vi "AlGaInPAs_prep_run_disc_v04.vi"(2 "Debug Mode":bool, 3 "Elapsed Time(s)":dbl, 4 "State":enum16{"Edit", "Start", "Run", "End", "Idle"}(ring), 5 "Argument List In":string[](array[string])) -> (0 "Status Out":string, 1 "Argument List Out":string[](array[string]))   [LabVIEW 2011]
panel:
  out "total time":dbl
  out "is OK?":bool
  out "Run started?":bool
  out "AsH3?":bool
  out "PH3?":bool
  out "In?":bool
  out "Ga?":bool
  out "Al?":bool
  in  "Prep As":bool caption="Pre-run"
  in  "Prep P":bool caption="Pre-run"
  in  "Prep In":bool caption="Pre-run"
  in  "Prep Ga":bool caption="Pre-run"
  in  "run_time":dbl caption="run time (s)"
  in  "prep_time":dbl caption="pre-run time (s)"
  in  "Prep Al":bool caption="Pre-run"
  in  "Run As":bool caption="Run"
  in  "AsH3 Flow":dbl caption="AsH3 Flow (0-10 sccm)" format="%.2f"
  in  "P Flow":dbl caption="P Flow (0-100 sccm)" format="%.2f"
  in  "Run P":bool caption="Run"
  in  "In Flow":dbl caption="In Flow (0-100 sscm)" format="%.2f"
  in  "Run In":bool caption="Run"
  in  "Run Ga":bool caption="Run"
  in  "Ga Flow":dbl caption="Ga Flow (0-10 sscm)" format="%.2f"
  in  "Run Al":bool caption="Run"
  in  "Al Flow":dbl caption="Al Flow (0-100 sscm)" format="%.2f"
  in  "Cancel":bool
  in  "OK":bool
  out "tTotal(s) 2":dbl
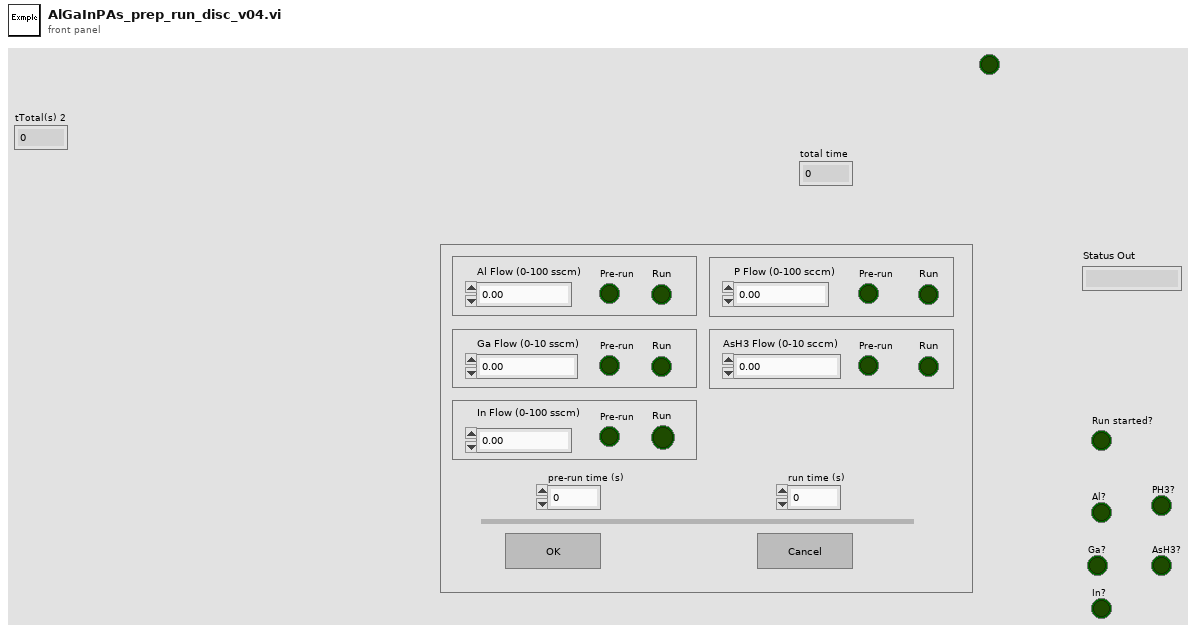
[diagram p1: front panel]
types:
  T1 = enum16{"Discrete", "Continuous", "Instantaneous"}
  T2 = enum32{"Invalid", "Default", "Floating", "Floating/Auto-Hide", "Modal"}
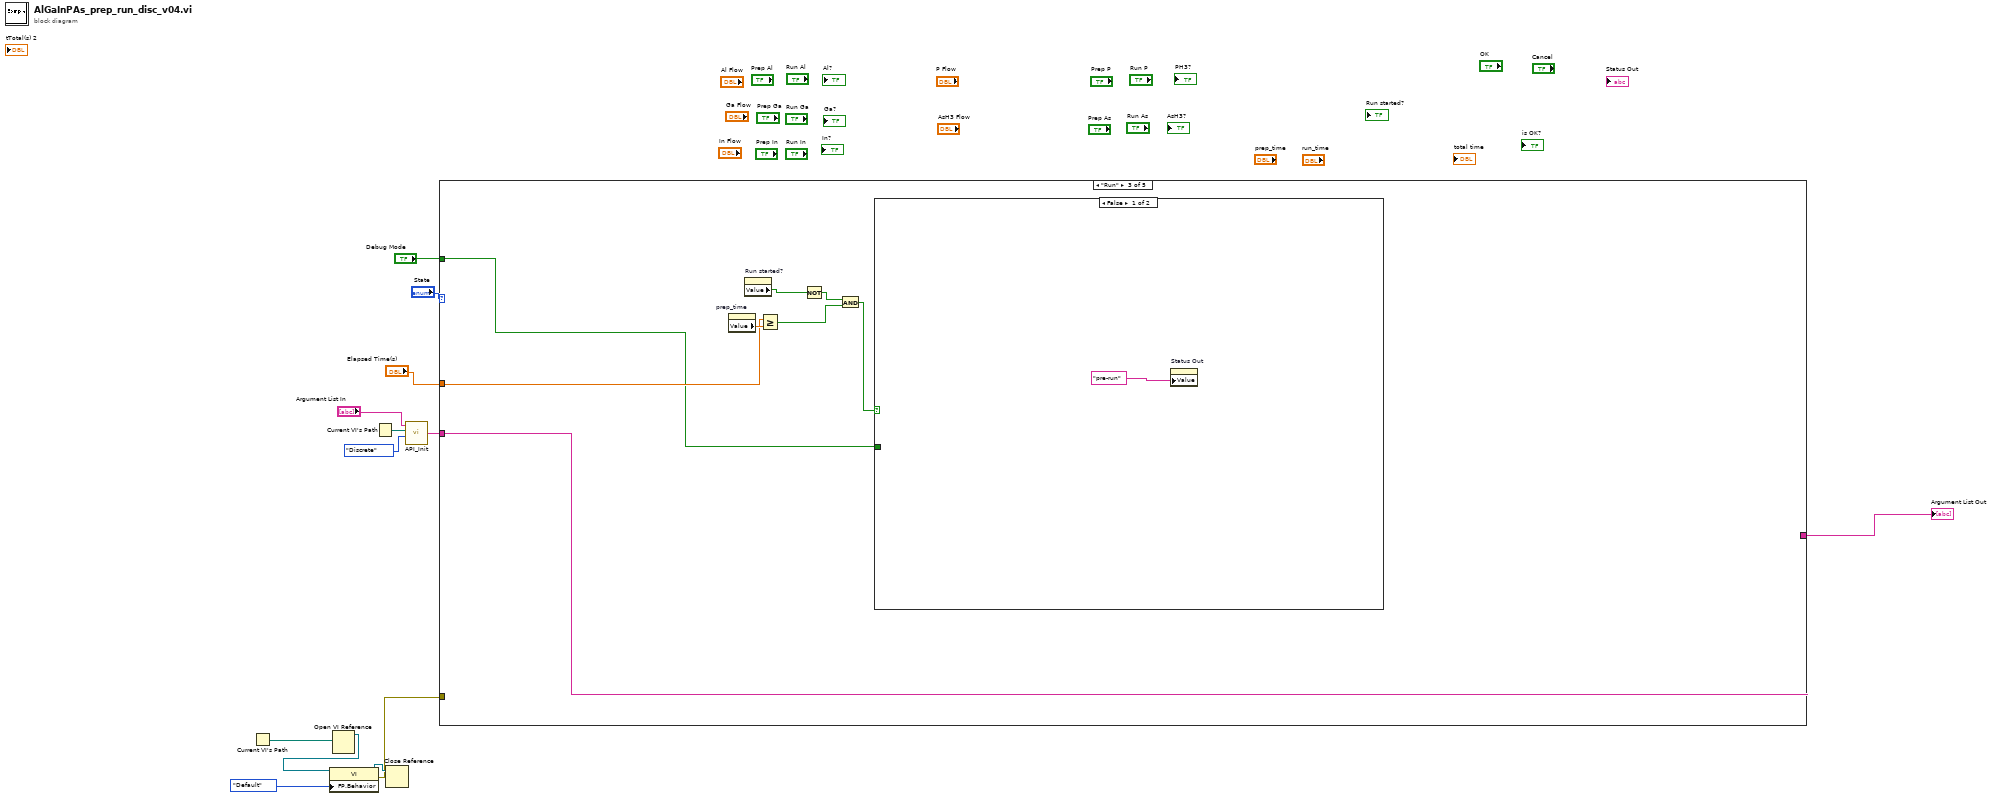
[diagram p0: block diagram]
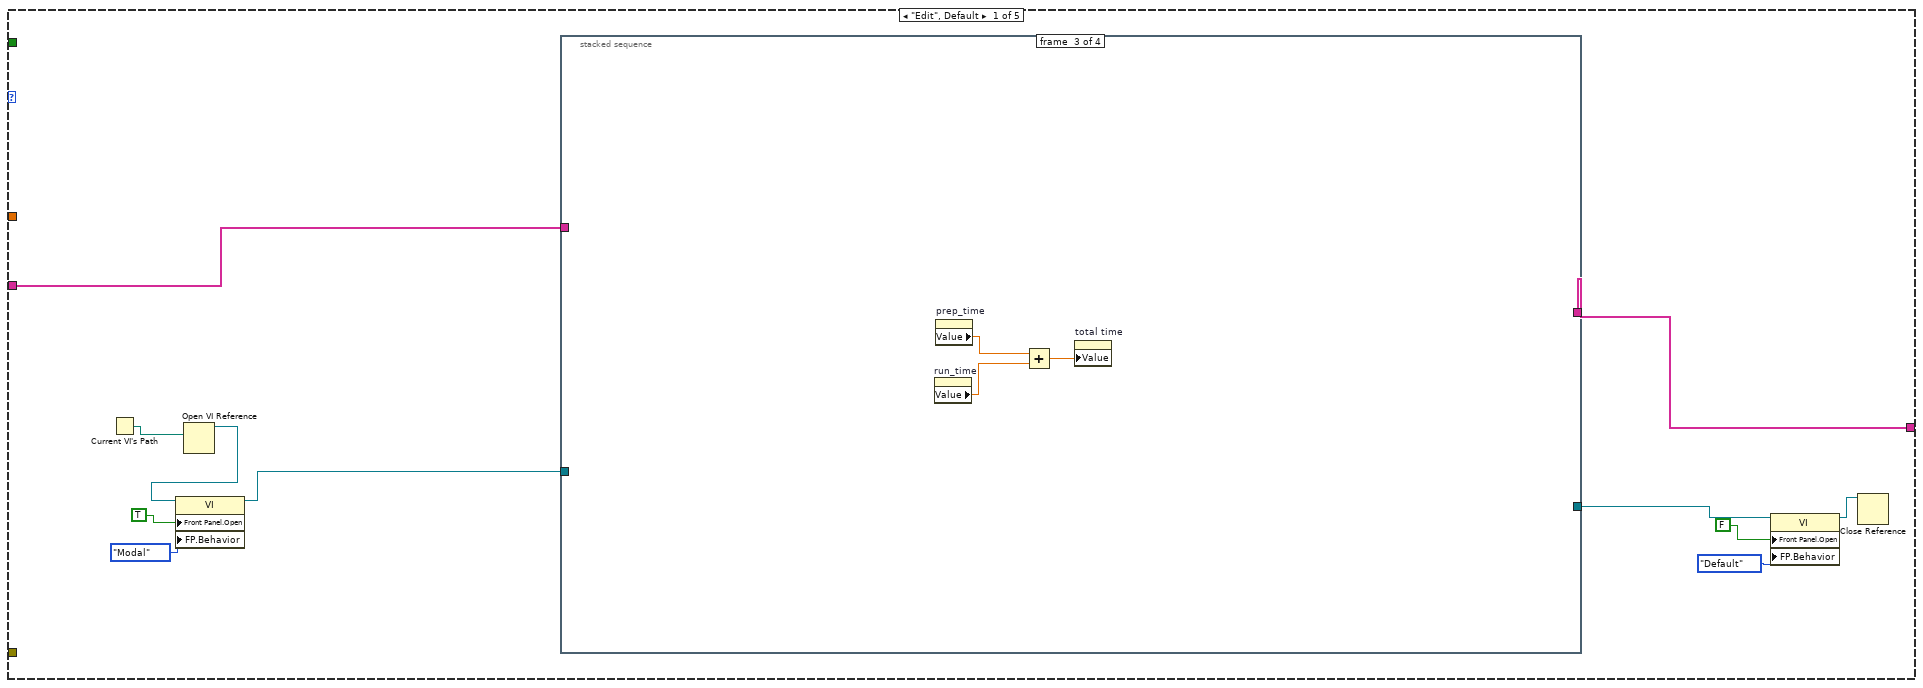
[diagram p2: hidden frame]
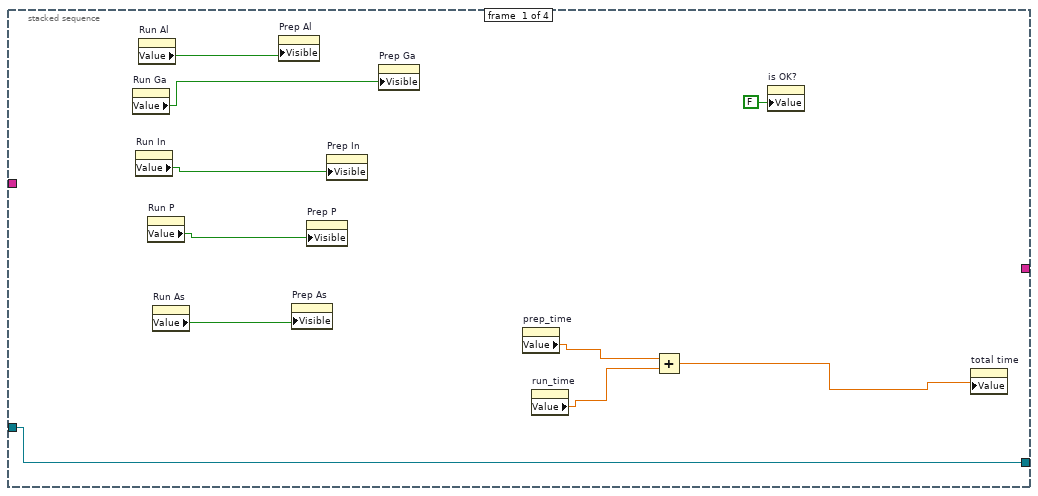
[diagram p3: hidden frame]
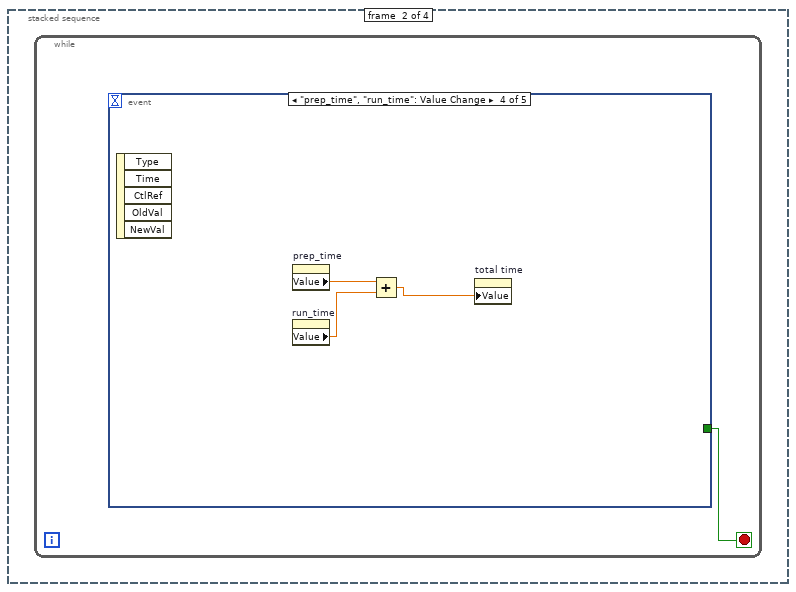
[diagram p4: hidden frame]
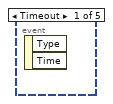
[diagram p5: hidden frame]
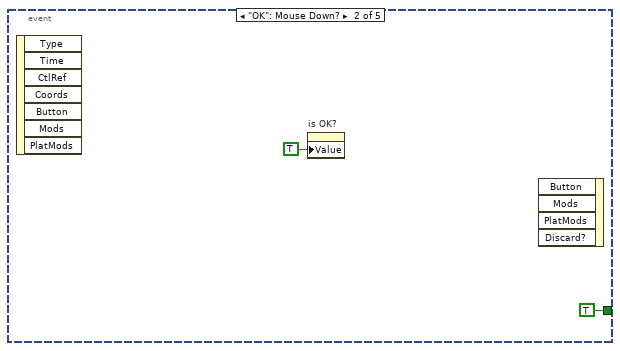
[diagram p6: hidden frame]
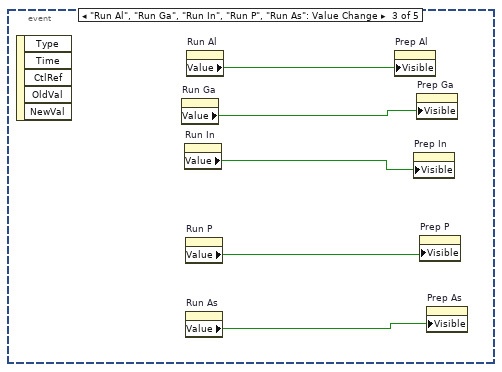
[diagram p7: hidden frame]
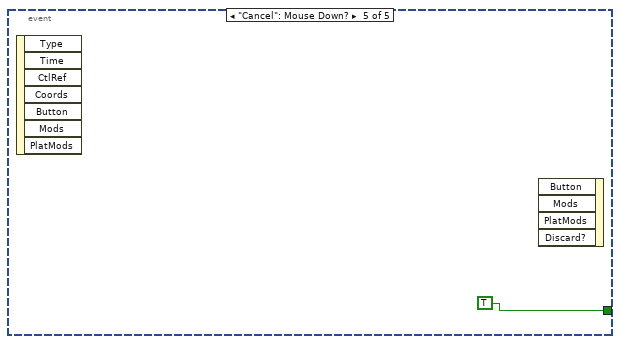
[diagram p8: hidden frame]
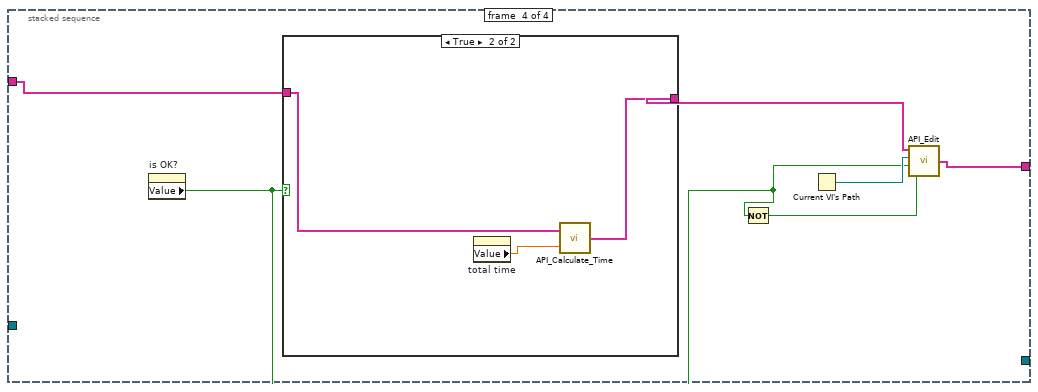
[diagram p9: hidden frame]
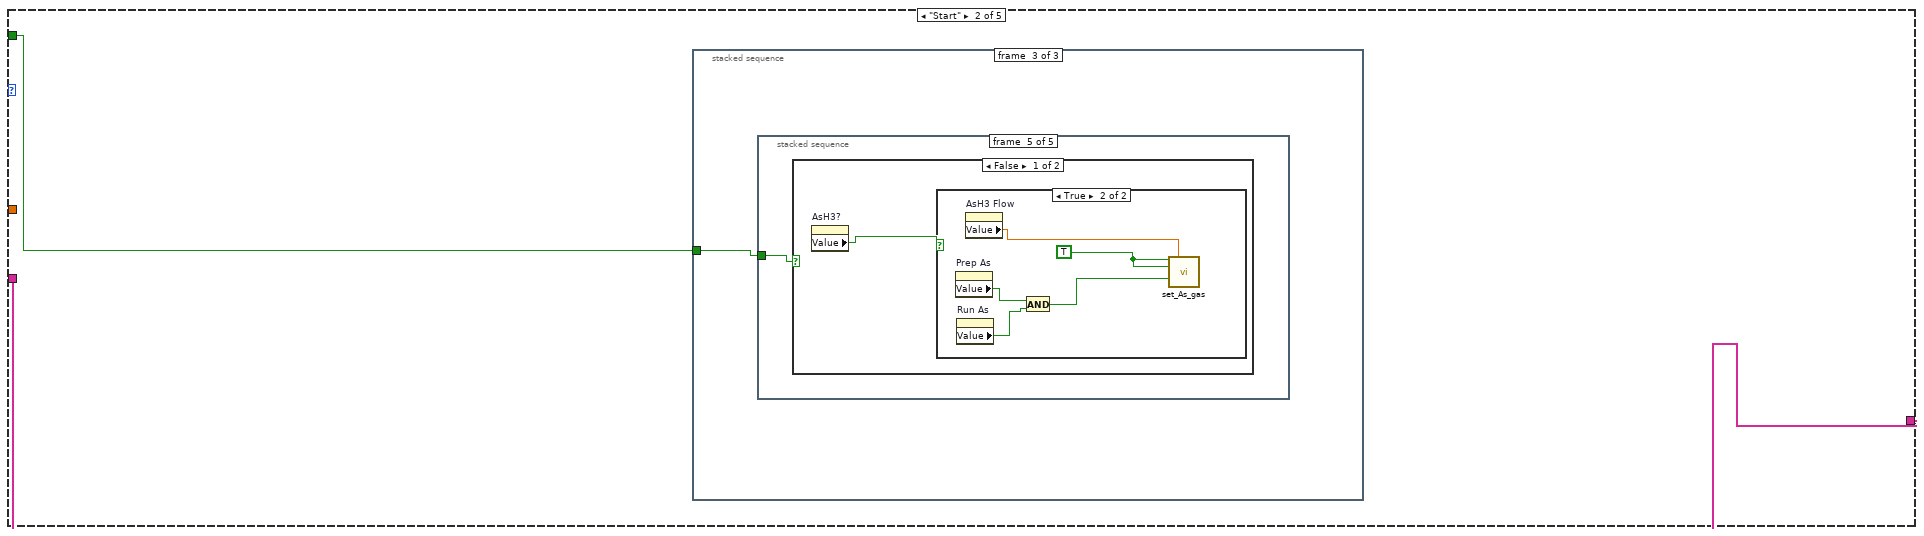
[diagram p11: hidden frame]
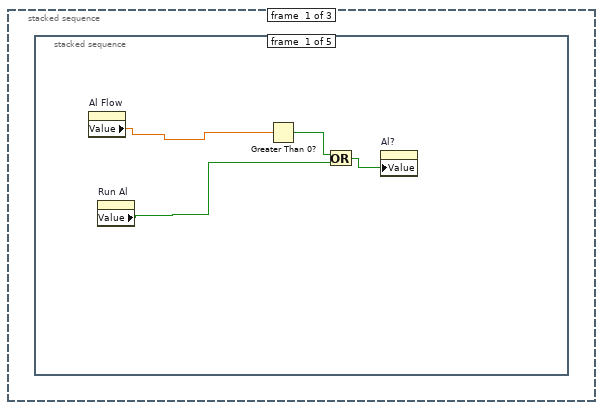
[diagram p12: hidden frame]
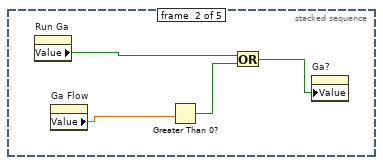
[diagram p13: hidden frame]
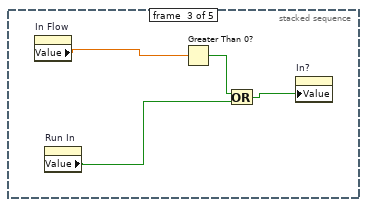
[diagram p14: hidden frame]
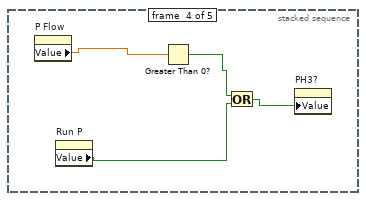
[diagram p15: hidden frame]
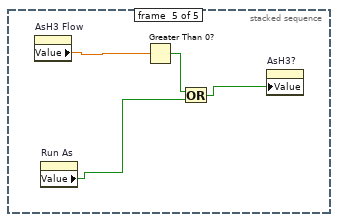
[diagram p16: hidden frame]
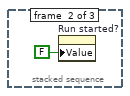
[diagram p17: hidden frame]
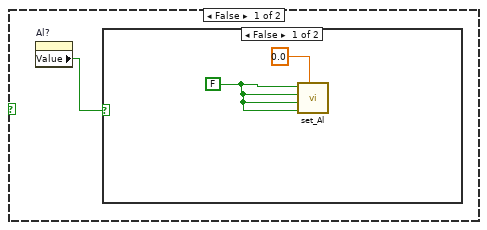
[diagram p19: hidden frame]
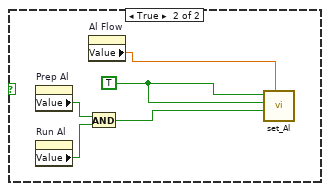
[diagram p20: hidden frame]
diagram:
  n1 = Current VI's Path() -> (path=w9:path)
  n2 = Open VI Reference(vi path=w9) -> (vi reference=w8:refnum<vi>)  [unwired: 1 in, 5 out]
  n3 = property class="VI"(reference=w8, "FP.Behavior"=T2."Default" ("Front Panel Window:Behavior")) -> (reference out=w6:refnum<vi>, error out=w5:errorcluster)  [unwired: 1 in]
  n4 = Current VI's Path() -> (path=w4:path)
  n5 = Close Reference(reference=w6) -> ()  [unwired: 1 in, 1 out]
  n6 = call "API_Init.vi"("API Mode"=T1."Discrete", "VI Path"=w4, "Argument List In"="Argument List In") -> ("Argument List Out"=w1:string[])  [unwired: 1 in]
  n7 = case shown="\"Run\"" "State" {
    tunnel: "Debug Mode" -> [_ w60 w134 _ _]
    tunnel: "Elapsed Time(s)" -> [_ _ w135 _ _]
    tunnel: w1 -> [w15 w61 w137 w179 w180]
    tunnel: [w14 w61 w137 w179 w180] -> w10
    tunnel: w5 -> [_ _ _ _ _]
    frame "Edit", Default {
      n8 = Current VI's Path() -> (path=w20:path)
      n9 = Open VI Reference(vi path=w20) -> (vi reference=w19:refnum<vi>)  [unwired: 1 in, 5 out]
      n10 = property class="VI"(reference=w19, "Front Panel.Open"=TRUE ("Front Panel Window:Open"), "FP.Behavior"=T2."Modal" ("Front Panel Window:Behavior")) -> (reference out=w18:refnum<vi>)  [unwired: 1 in, 1 out]
      n11 = stacked-sequence {
        tunnel: w15 -> [_ _ _ w53]
        tunnel: w18 -> [w32 _ _ _]
        tunnel: [w32 _ _ _] -> w22
        tunnel: [_ _ _ w51] -> w14
        frame #0 {
          n12 = property on="Run Ga" class="Bool (strict)"() -> ("Value"=w28:bool)  [unwired: 2 in, 2 out]
          n13 = property on="Run In" class="Bool (strict)"() -> ("Value"=w27:bool)  [unwired: 2 in, 2 out]
          n14 = property on="Run Al" class="Bool (strict)"() -> ("Value"=w29:bool)  [unwired: 2 in, 2 out]
          n15 = property on="Run P" class="Bool (strict)"() -> ("Value"=w26:bool)  [unwired: 2 in, 2 out]
          n16 = property on="Run As" class="Bool (strict)"() -> ("Value"=w25:bool)  [unwired: 2 in, 2 out]
          n17 = property on="Prep Al" class="Bool (strict)"("Visible"=w29) -> ()  [unwired: 2 in, 2 out]
          n18 = property on="Prep As" class="Bool (strict)"("Visible"=w25) -> ()  [unwired: 2 in, 2 out]
          n19 = property on="Prep P" class="Bool (strict)"("Visible"=w26) -> ()  [unwired: 2 in, 2 out]
          n20 = property on="Prep In" class="Bool (strict)"("Visible"=w27) -> ()  [unwired: 2 in, 2 out]
          n21 = property on="Prep Ga" class="Bool (strict)"("Visible"=w28) -> ()  [unwired: 2 in, 2 out]
          n22 = property on="prep_time" class="DigNum (strict)"() -> ("Value"=w34:dbl)  [unwired: 2 in, 2 out]
          n23 = property on="run_time" class="DigNum (strict)"() -> ("Value"=w33:dbl)  [unwired: 2 in, 2 out]
          n24 = Add(x=w34, y=w33) -> (x+y=w30:dbl)
          n25 = property on="is OK?" class="Bool (strict)"("Value"=FALSE ("is OK?")) -> ()  [unwired: 2 in, 2 out]
          n26 = property on="total time" class="DigNum (strict)"("Value"=w30) -> ()  [unwired: 2 in, 2 out]
        }
        frame #1 {
          n27 = while {
            stop <- w35 stop-if-true
            n28 = event shown="[3] \"prep_time\", \"run_time\": Value Change" {
              selector: _ -> [_ _ _ _ _]
              dyn-events: _ -> [_ _ _ _ _]
              timeout: _ -> [_ _ _ _ _]
              tunnel: [_ TRUE _ _ TRUE] -> w35
              event Timeout {
                n29 = event-data() -> ()  [unwired: 1 in, 2 out]
              }
              event "OK": Mouse Down? {
                n30 = event-data() -> ()  [unwired: 1 in, 7 out]
                n31 = property on="is OK?" class="Bool (strict)"("Value"=TRUE ("is OK?")) -> ()  [unwired: 2 in, 2 out]
                n32 = event-data() -> ()  [unwired: 5 in, 1 out]
              }
              event "Run Al", "Run Ga", "Run In", "Run P", "Run As": Value Change {
                n33 = event-data() -> ()  [unwired: 1 in, 5 out]
                n34 = property on="Run Ga" class="Bool (strict)"() -> ("Value"=w41:bool)  [unwired: 2 in, 2 out]
                n35 = property on="Run In" class="Bool (strict)"() -> ("Value"=w40:bool)  [unwired: 2 in, 2 out]
                n36 = property on="Run P" class="Bool (strict)"() -> ("Value"=w39:bool)  [unwired: 2 in, 2 out]
                n37 = property on="Run As" class="Bool (strict)"() -> ("Value"=w38:bool)  [unwired: 2 in, 2 out]
                n38 = property on="Run Al" class="Bool (strict)"() -> ("Value"=w42:bool)  [unwired: 2 in, 2 out]
                n39 = property on="Prep Al" class="Bool (strict)"("Visible"=w42) -> ()  [unwired: 2 in, 2 out]
                n40 = property on="Prep In" class="Bool (strict)"("Visible"=w40) -> ()  [unwired: 2 in, 2 out]
                n41 = property on="Prep Ga" class="Bool (strict)"("Visible"=w41) -> ()  [unwired: 2 in, 2 out]
                n42 = property on="Prep P" class="Bool (strict)"("Visible"=w39) -> ()  [unwired: 2 in, 2 out]
                n43 = property on="Prep As" class="Bool (strict)"("Visible"=w38) -> ()  [unwired: 2 in, 2 out]
              }
              event "prep_time", "run_time": Value Change {
                n44 = event-data() -> ()  [unwired: 1 in, 5 out]
                n45 = property on="prep_time" class="DigNum (strict)"() -> ("Value"=w45:dbl)  [unwired: 2 in, 2 out]
                n46 = property on="run_time" class="DigNum (strict)"() -> ("Value"=w44:dbl)  [unwired: 2 in, 2 out]
                n47 = Add(x=w45, y=w44) -> (x+y=w43:dbl)
                n48 = property on="total time" class="DigNum (strict)"("Value"=w43) -> ()  [unwired: 2 in, 2 out]
              }
              event "Cancel": Mouse Down? {
                n49 = event-data() -> ()  [unwired: 1 in, 7 out]
                n50 = event-data() -> ()  [unwired: 5 in, 1 out]
              }
            }
          }
        }
        frame #2 {
          n51 = property on="run_time" class="DigNum (strict)"() -> ("Value"=w48:dbl)  [unwired: 2 in, 2 out]
          n52 = property on="prep_time" class="DigNum (strict)"() -> ("Value"=w47:dbl)  [unwired: 2 in, 2 out]
          n53 = Add(x=w47, y=w48) -> (x+y=w49:dbl)
          n54 = property on="total time" class="DigNum (strict)"("Value"=w49) -> ()  [unwired: 2 in, 2 out]
        }
        frame #3 {
          n55 = property on="is OK?" class="Bool (strict)"() -> ("Value"=w50:bool)  [unwired: 2 in, 2 out]
          n56 = case shown="True" w50 {
            tunnel: w53 -> [w56 w58]
            tunnel: [w56 w57] -> w52
            frame False {
            }
            frame True {
              n57 = property on="total time" class="DigNum (strict)"() -> ("Value"=w59:dbl)  [unwired: 2 in, 2 out]
              n58 = call "API_Calculate_Time.vi"("Time"=w59, "Argument List In"=w58) -> ("Argument List Out"=w57:string[])
            }
          }
          n59 = Not(x=w50) -> (.not. x?=w55:bool)
          n60 = Current VI's Path() -> (path=w54:path)
          n61 = call "API_Edit.vi"("Cancel"=w55, "OK"=w50, "VI Path"=w54, "Argument List In"=w52) -> ("Argument List Out"=w51:string[])
        }
      }
      n62 = property class="VI"(reference=w22, "Front Panel.Open"=FALSE ("Front Panel Window:Open"), "FP.Behavior"=T2."Default" ("Front Panel Window:Behavior")) -> (reference out=w23:refnum<vi>)  [unwired: 1 in, 1 out]
      n63 = Close Reference(reference=w23) -> ()  [unwired: 1 in, 1 out]
    }
    frame "Start" {
      n64 = stacked-sequence {
        tunnel: w60 -> [_ _ w83]
        frame #0 {
          n65 = stacked-sequence {
            frame #0 {
              n66 = property on="Al Flow" class="DigNum (strict)"() -> ("Value"=w64:dbl)  [unwired: 2 in, 2 out]
              n67 = property on="Run Al" class="Bool (strict)"() -> ("Value"=w63:bool)  [unwired: 2 in, 2 out]
              n68 = Greater Than 0?(x=w64) -> (x > 0?=w65:bool)
              n69 = Or(x=w65, y=w63) -> (x .or. y?=w62:bool)
              n70 = property on="Al?" class="Bool (strict)"("Value"=w62) -> ()  [unwired: 2 in, 2 out]
            }
            frame #1 {
              n71 = property on="Run Ga" class="Bool (strict)"() -> ("Value"=w67:bool)  [unwired: 2 in, 2 out]
              n72 = property on="Ga Flow" class="DigNum (strict)"() -> ("Value"=w68:dbl)  [unwired: 2 in, 2 out]
              n73 = Greater Than 0?(x=w68) -> (x > 0?=w69:bool)
              n74 = Or(x=w67, y=w69) -> (x .or. y?=w66:bool)
              n75 = property on="Ga?" class="Bool (strict)"("Value"=w66) -> ()  [unwired: 2 in, 2 out]
            }
            frame #2 {
              n76 = property on="In Flow" class="DigNum (strict)"() -> ("Value"=w71:dbl)  [unwired: 2 in, 2 out]
              n77 = property on="Run In" class="Bool (strict)"() -> ("Value"=w72:bool)  [unwired: 2 in, 2 out]
              n78 = Greater Than 0?(x=w71) -> (x > 0?=w73:bool)
              n79 = Or(x=w73, y=w72) -> (x .or. y?=w70:bool)
              n80 = property on="In?" class="Bool (strict)"("Value"=w70) -> ()  [unwired: 2 in, 2 out]
            }
            frame #3 {
              n81 = property on="P Flow" class="DigNum (strict)"() -> ("Value"=w76:dbl)  [unwired: 2 in, 2 out]
              n82 = property on="Run P" class="Bool (strict)"() -> ("Value"=w75:bool)  [unwired: 2 in, 2 out]
              n83 = Greater Than 0?(x=w76) -> (x > 0?=w77:bool)
              n84 = Or(x=w77, y=w75) -> (x .or. y?=w74:bool)
              n85 = property on="PH3?" class="Bool (strict)"("Value"=w74) -> ()  [unwired: 2 in, 2 out]
            }
            frame #4 {
              n86 = property on="AsH3 Flow" class="DigNum (strict)"() -> ("Value"=w80:dbl)  [unwired: 2 in, 2 out]
              n87 = property on="Run As" class="Bool (strict)"() -> ("Value"=w79:bool)  [unwired: 2 in, 2 out]
              n88 = Greater Than 0?(x=w80) -> (x > 0?=w81:bool)
              n89 = Or(x=w81, y=w79) -> (x .or. y?=w78:bool)
              n90 = property on="AsH3?" class="Bool (strict)"("Value"=w78) -> ()  [unwired: 2 in, 2 out]
            }
          }
        }
        frame #1 {
          n91 = property on="Run started?" class="Bool (strict)"("Value"=FALSE ("Run started?")) -> ()  [unwired: 2 in, 2 out]
        }
        frame #2 {
          n92 = stacked-sequence {
            tunnel: w83 -> [w84 w93 w103 w112 w121]
            frame #0 {
              n93 = case shown="True" w84 {
                frame False {
                  n94 = property on="Al?" class="Bool (strict)"() -> ("Value"=w85:bool)  [unwired: 2 in, 2 out]
                  n95 = case shown="False" w85 {
                    frame False {
                      w86 = FALSE ("Al Active")
                      n96 = call "set_Al.vi"("Aluminum Flow"=0.0, "Al Remote"=w86, "Al Run"=w86, "Al Bubbler"=w86, "Al Active"=w86) -> ()  [unwired: 5 out]
                    }
                    frame True {
                      w92 = TRUE ("Al Active")
                      n97 = property on="Prep Al" class="Bool (strict)"() -> ("Value"=w90:bool)  [unwired: 2 in, 2 out]
                      n98 = property on="Run Al" class="Bool (strict)"() -> ("Value"=w89:bool)  [unwired: 2 in, 2 out]
                      n99 = property on="Al Flow" class="DigNum (strict)"() -> ("Value"=w91:dbl)  [unwired: 2 in, 2 out]
                      n100 = And(x=w90, y=w89) -> (x .and. y?=w88:bool)
                      n101 = call "set_Al.vi"("Aluminum Flow"=w91, "Al Run"=w88, "Al Bubbler"=w92, "Al Active"=w92) -> ()  [unwired: 1 in, 5 out]
                    }
                  }
                }
                frame True {
                }
              }
            }
            frame #1 {
              n102 = case shown="False" w93 {
                frame False {
                  n103 = property on="Ga?" class="Bool (strict)"() -> ("Value"=w94:bool)  [unwired: 2 in, 2 out]
                  n104 = case shown="True" w94 {
                    frame False {
                      w96 = FALSE ("Ga Active")
                      w95 = 0.0 ("Ga Flow 1")
                      n105 = call "set_Ga.vi"("Ga Active"=w96, "Ga Flow 3"=w95, "Ga Flow 2"=w95, "Ga Flow 1"=w95, "Ga Bubbler"=w96, "Ga H2 Dilute"=w96, "Ga Run"=w96, "Ga Remote"=w96) -> ()  [unwired: 8 out]
                    }
                    frame True {
                      w102 = TRUE ("Ga Active")
                      n106 = property on="Prep Ga" class="Bool (strict)"() -> ("Value"=w99:bool)  [unwired: 2 in, 2 out]
                      n107 = property on="Run Ga" class="Bool (strict)"() -> ("Value"=w98:bool)  [unwired: 2 in, 2 out]
                      n108 = And(x=w99, y=w98) -> (x .and. y?=w97:bool)
                      n109 = property on="Ga Flow" class="DigNum (strict)"() -> ("Value"=w100:dbl)  [unwired: 2 in, 2 out]
                      n110 = call "set_Ga_dilut_cond.vi"("Ga flow (0-10 sccm)"=w100, "fDilution"=0.0, "Run"=w97, "Bubbler In"=w102, "Active"=w102) -> ()
                    }
                  }
                }
                frame True {
                }
              }
            }
            frame #2 {
              n111 = case shown="False" w103 {
                frame False {
                  n112 = property on="In?" class="Bool (strict)"() -> ("Value"=w104:bool)  [unwired: 2 in, 2 out]
                  n113 = case shown="True" w104 {
                    frame False {
                      w106 = FALSE ("In Remote")
                      n114 = call "set_In.vi"("Indium Flow"=0.0, "In Remote"=w106, "In Run"=w106, "In Bubbler"=w106, "In Active"=w106) -> ()  [unwired: 5 out]
                    }
                    frame True {
                      w111 = TRUE ("In Run")
                      n115 = property on="Run In" class="Bool (strict)"() -> ("Value"=w108:bool)  [unwired: 2 in, 2 out]
                      n116 = property on="Prep In" class="Bool (strict)"() -> ("Value"=w109:bool)  [unwired: 2 in, 2 out]
                      n117 = And(x=w109, y=w108) -> (x .and. y?=w107:bool)
                      n118 = property on="In Flow" class="DigNum (strict)"() -> ("Value"=w110:dbl)  [unwired: 2 in, 2 out]
                      n119 = call "set_In.vi"("Indium Flow"=w110, "In Run"=w107, "In Bubbler"=w111, "In Active"=w111) -> ()  [unwired: 1 in, 5 out]
                    }
                  }
                }
                frame True {
                }
              }
            }
            frame #3 {
              n120 = case shown="False" w112 {
                frame False {
                  n121 = property on="PH3?" class="Bool (strict)"() -> ("Value"=w113:bool)  [unwired: 2 in, 2 out]
                  n122 = case shown="True" w113 {
                    frame False {
                      w114 = FALSE ("P_Gas Active")
                      n123 = call "set_P_gas.vi"("P_Gas Active"=w114, "P_Gas Flow"=0.0, "P_Gas In"=w114, "P_Gas H2 In"=w114, "P_Gas Run"=w114, "P_Gas Remote"=w114) -> ()  [unwired: 10 out]
                    }
                    frame True {
                      w120 = TRUE ("P_Gas Active")
                      n124 = property on="P Flow" class="DigNum (strict)"() -> ("Value"=w119:dbl)  [unwired: 2 in, 2 out]
                      n125 = property on="Prep P" class="Bool (strict)"() -> ("Value"=w118:bool)  [unwired: 2 in, 2 out]
                      n126 = property on="Run P" class="Bool (strict)"() -> ("Value"=w117:bool)  [unwired: 2 in, 2 out]
                      n127 = And(x=w118, y=w117) -> (x .and. y?=w116:bool)
                      n128 = call "set_P_gas.vi"("P_Gas Active"=w120, "P_Gas Flow"=w119, "P_Gas In"=w120, "P_Gas Run"=w116) -> ()  [unwired: 2 in, 10 out]
                    }
                  }
                }
                frame True {
                }
              }
            }
            frame #4 {
              n129 = case shown="False" w121 {
                frame False {
                  n130 = property on="AsH3?" class="Bool (strict)"() -> ("Value"=w122:bool)  [unwired: 2 in, 2 out]
                  n131 = case shown="True" w122 {
                    frame False {
                      w123 = FALSE ("As_Gas Active")
                      n132 = call "set_As_gas.vi"("As_Gas Active"=w123, "As_Gas Flow"=0.0, "As_Gas In"=w123, "As_Gas H2"=w123, "As_Gas Run"=w123, "As_Gas Remote"=w123) -> ()  [unwired: 10 in]
                    }
                    frame True {
                      w129 = TRUE ("As_Gas Active")
                      n133 = property on="Prep As" class="Bool (strict)"() -> ("Value"=w126:bool)  [unwired: 2 in, 2 out]
                      n134 = property on="Run As" class="Bool (strict)"() -> ("Value"=w127:bool)  [unwired: 2 in, 2 out]
                      n135 = property on="AsH3 Flow" class="DigNum (strict)"() -> ("Value"=w128:dbl)  [unwired: 2 in, 2 out]
                      n136 = And(x=w126, y=w127) -> (x .and. y?=w125:bool)
                      n137 = call "set_As_gas.vi"("As_Gas Active"=w129, "As_Gas Flow"=w128, "As_Gas In"=w129, "As_Gas Run"=w125) -> ()  [unwired: 12 in]
                    }
                  }
                }
                frame True {
                }
              }
            }
          }
        }
      }
    }
    frame "Run" {
      n138 = property on="prep_time" class="DigNum (strict)"() -> ("Value"=w136:dbl)  [unwired: 2 in, 2 out]
      n139 = property on="Run started?" class="Bool (strict)"() -> ("Value"=w131:bool)  [unwired: 2 in, 2 out]
      n140 = Greater Or Equal?(x=w135, y=w136) -> (x >= y?=w133:bool)
      n141 = Not(x=w131) -> (.not. x?=w130:bool)
      n142 = And(x=w130, y=w133) -> (x .and. y?=w132:bool)
      n143 = case shown="False" w132 {
        tunnel: w134 -> [_ w139]
        frame False {
          n144 = property on="Status Out" class="Str"("Value"="pre-run" ("Status Out")) -> ()  [unwired: 2 in, 2 out]
        }
        frame True {
          n145 = stacked-sequence {
            tunnel: w139 -> [w140]
            frame #0 {
              n146 = stacked-sequence {
                tunnel: w140 -> [w141 w148 w156 w163 w170 _]
                frame #0 {
                  n147 = case shown="False" w141 {
                    frame False {
                      n148 = property on="Al?" class="Bool (strict)"() -> ("Value"=w142:bool)  [unwired: 2 in, 2 out]
                      n149 = case shown="True" w142 {
                        frame False {
                          w143 = FALSE ("Al Active")
                          n150 = call "set_Al.vi"("Aluminum Flow"=0.0, "Al Remote"=w143, "Al Run"=w143, "Al Bubbler"=w143, "Al Active"=w143) -> ()  [unwired: 5 out]
                        }
                        frame True {
                          w147 = TRUE ("Al Active")
                          n151 = property on="Al Flow" class="DigNum (strict)"() -> ("Value"=w146:dbl)  [unwired: 2 in, 2 out]
                          n152 = property on="Run Al" class="Bool (strict)"() -> ("Value"=w145:bool)  [unwired: 2 in, 2 out]
                          n153 = call "set_Al.vi"("Aluminum Flow"=w146, "Al Run"=w145, "Al Bubbler"=w147, "Al Active"=w147) -> ()  [unwired: 1 in, 5 out]
                        }
                      }
                    }
                    frame True {
                    }
                  }
                }
                frame #1 {
                  n154 = case shown="False" w148 {
                    frame False {
                      n155 = property on="Ga?" class="Bool (strict)"() -> ("Value"=w149:bool)  [unwired: 2 in, 2 out]
                      n156 = case shown="True" w149 {
                        frame False {
                          w151 = FALSE ("Ga Active")
                          w150 = 0.0 ("Ga Flow 1")
                          n157 = call "set_Ga.vi"("Ga Active"=w151, "Ga Flow 3"=w150, "Ga Flow 2"=w150, "Ga Flow 1"=w150, "Ga Bubbler"=w151, "Ga H2 Dilute"=w151, "Ga Run"=w151, "Ga Remote"=w151) -> ()  [unwired: 8 out]
                        }
                        frame True {
                          w155 = TRUE ("Ga Active")
                          n158 = property on="Ga Flow" class="DigNum (strict)"() -> ("Value"=w152:dbl)  [unwired: 2 in, 2 out]
                          n159 = property on="Run Ga" class="Bool (strict)"() -> ("Value"=w153:bool)  [unwired: 2 in, 2 out]
                          n160 = call "set_Ga_dilut_cond.vi"("Ga flow (0-10 sccm)"=w152, "fDilution"=0.0, "Run"=w153, "Bubbler In"=w155, "Active"=w155) -> ()
                        }
                      }
                    }
                    frame True {
                    }
                  }
                }
                frame #2 {
                  n161 = case shown="False" w156 {
                    frame False {
                      n162 = property on="In?" class="Bool (strict)"() -> ("Value"=w157:bool)  [unwired: 2 in, 2 out]
                      n163 = case shown="True" w157 {
                        frame False {
                          w159 = FALSE ("In Remote")
                          n164 = call "set_In.vi"("Indium Flow"=0.0, "In Remote"=w159, "In Run"=w159, "In Bubbler"=w159, "In Active"=w159) -> ()  [unwired: 5 out]
                        }
                        frame True {
                          w162 = TRUE ("In Run")
                          n165 = property on="Run In" class="Bool (strict)"() -> ("Value"=w160:bool)  [unwired: 2 in, 2 out]
                          n166 = property on="In Flow" class="DigNum (strict)"() -> ("Value"=w161:dbl)  [unwired: 2 in, 2 out]
                          n167 = call "set_In.vi"("Indium Flow"=w161, "In Run"=w160, "In Bubbler"=w162, "In Active"=w162) -> ()  [unwired: 1 in, 5 out]
                        }
                      }
                    }
                    frame True {
                    }
                  }
                }
                frame #3 {
                  n168 = case shown="False" w163 {
                    frame False {
                      n169 = property on="PH3?" class="Bool (strict)"() -> ("Value"=w164:bool)  [unwired: 2 in, 2 out]
                      n170 = case shown="False" w164 {
                        frame False {
                          w165 = FALSE ("P_Gas Active")
                          n171 = call "set_P_gas.vi"("P_Gas Active"=w165, "P_Gas Flow"=0.0, "P_Gas In"=w165, "P_Gas H2 In"=w165, "P_Gas Run"=w165, "P_Gas Remote"=w165) -> ()  [unwired: 10 out]
                        }
                        frame True {
                          w169 = TRUE ("P_Gas Active")
                          n172 = property on="P Flow" class="DigNum (strict)"() -> ("Value"=w168:dbl)  [unwired: 2 in, 2 out]
                          n173 = property on="Run P" class="Bool (strict)"() -> ("Value"=w167:bool)  [unwired: 2 in, 2 out]
                          n174 = call "set_P_gas.vi"("P_Gas Active"=w169, "P_Gas Flow"=w168, "P_Gas In"=w169, "P_Gas Run"=w167) -> ()  [unwired: 2 in, 10 out]
                        }
                      }
                    }
                    frame True {
                    }
                  }
                }
                frame #4 {
                  n175 = case shown="False" w170 {
                    frame False {
                      n176 = property on="AsH3?" class="Bool (strict)"() -> ("Value"=w171:bool)  [unwired: 2 in, 2 out]
                      n177 = case shown="False" w171 {
                        frame False {
                          w172 = FALSE ("As_Gas Active")
                          n178 = call "set_As_gas.vi"("As_Gas Active"=w172, "As_Gas Flow"=0.0, "As_Gas In"=w172, "As_Gas H2"=w172, "As_Gas Run"=w172, "As_Gas Remote"=w172) -> ()  [unwired: 10 in]
                        }
                        frame True {
                          w175 = TRUE ("As_Gas Active")
                          n179 = property on="Run As" class="Bool (strict)"() -> ("Value"=w174:bool)  [unwired: 2 in, 2 out]
                          n180 = property on="AsH3 Flow" class="DigNum (strict)"() -> ("Value"=w176:dbl)  [unwired: 2 in, 2 out]
                          n181 = call "set_As_gas.vi"("As_Gas Active"=w175, "As_Gas Flow"=w176, "As_Gas In"=w175, "As_Gas Run"=w174) -> ()  [unwired: 12 in]
                        }
                      }
                    }
                    frame True {
                    }
                  }
                }
                frame #5 {
                  n182 = property on="Status Out" class="Str"("Value"="run started" ("Status Out")) -> ()  [unwired: 2 in, 2 out]
                  n183 = property on="Run started?" class="Bool (strict)"("Value"=TRUE ("Run started?")) -> ()  [unwired: 2 in, 2 out]
                }
              }
            }
          }
        }
      }
    }
    frame "End" {
    }
    frame "Idle" {
    }
  }
  "Argument List Out" <- w10
